vi "Get Transmit Period.vi"(8 "error in":errorcluster, 11 "label ref":T1 format="%.0x") -> (0 "error out":errorcluster, 2 "transmit period (us)":u32, 3 "label ref out":T1 format="%.0x")   [LabVIEW 2020, in "Ballard ARINC 429 Scripting.lvlib"]
uses:
  Ballard ARINC 429 Scripting.lvlib
  <vilib>/NI VeriStand/Custom Device API/Custom Device Item Ref.ctl
  Constants.vi
  <vilib>/NI VeriStand/Custom Device API/Get Item Property (U32).vi
  <vilib>/NI VeriStand/Custom Device API/Custom Device API.lvlib
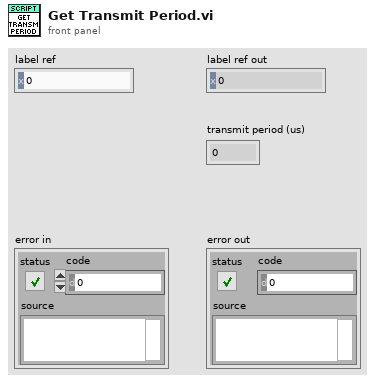
[diagram p1: front panel]
types:
  T1 = typedef "Custom Device API.lvlib/Custom Device Item Ref.ctl" = u64
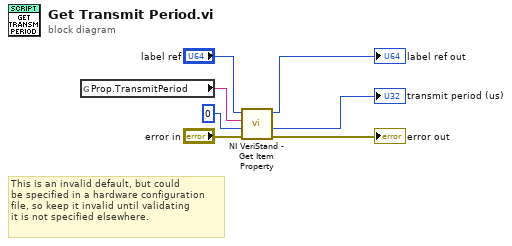
[diagram p0: block diagram]
diagram:
  # "This is an invalid default, but could\nbe specified in a hardware configuration\nfile, so keep it invalid until validating\nit is not specified elsewhere."
  n1 = global read "Constants.vi" "Prop.TransmitPeriod"() -> (w1:string)
  n2 = call-poly <vilib>:"NI VeriStand - Get Item Property.vi"("error in (no error)"="error in", "Default Value"=u32 0, "Property Name"=w1, "Item Ref in"="label ref") -> ("error out"=→"error out":errorcluster, "Value"=→"transmit period (us)":u32, "Item Ref out"=→"label ref out":T1)  [unwired: 4 in, 1 out]
